vi "PIDController_EnableContinousInput.vi"(9 "MaxInput":dbl, 10 "MinInput":dbl, 11 "in PID_CONTROLLER":T1={"Kp"=0.0, "Ki"=0.0, "Kd"=0.0, "Period"=0.0, "Max_Integral"=0.0, "Min_Integral"=0.0, "Max_Input"=0.0, "Min_Input"=0.0, "Continuous"=FALSE, "PositionError"=0.0, "VelocityError"=0.0, "PrevError"=0.0, "TotalError"=0.0, "PositionTolerance"=0.0, "VelocityTolerance"=0.0, "SetPoint"=0.0, "Kf"=0.0, "Prev_Deriv"=0.0, "Prev_Deriv 2"=0.0, "DerivativeFilter"=FALSE, "Min_Output"=-9.99e+35, "Max_Output"=9.9e+35, "Prev_F_P"=0.0, "Prev_F_P_2"=0.0, "AntiWindupActive"=FALSE, "Measurement"=0.0, "IntegralZone"=9.9e+30} {"IntegralZone" format="%16_6e"; "Measurement" format="%16_6e"; "Prev_F_P_2" format="%16_6e"; "Prev_F_P" format="%16_6e"; "Max_Output" format="%16_6e"; "Min_Output" format="%16_6e"; "Prev_Deriv 2" format="%16_6e"; "Prev_Deriv" format="%16_6e"; "Kf" format="%16_6e"; "SetPoint" format="%16_6e"; "VelocityTolerance" format="%16_6e"; "PositionTolerance" format="%16_6e"; "TotalError" format="%16_6e"; "PrevError" format="%16_6e"; "VelocityError" format="%16_6e"; "PositionError" format="%16_6e"; "Min_Input" format="%16_6e"; "Max_Input" format="%16_6e"; "Min_Integral" format="%16_6e"; "Max_Integral" format="%16_6e"; "Period" format="%16_6e"; "Kd" format="%16_6e"; "Ki" format="%16_6e"; "Kp" format="%16_6e"}) -> (3 "out PID_CONTROLLER":T1={"Kp"=0.0, "Ki"=0.0, "Kd"=0.0, "Period"=0.0, "Max_Integral"=0.0, "Min_Integral"=0.0, "Max_Input"=0.0, "Min_Input"=0.0, "Continuous"=FALSE, "PositionError"=0.0, "VelocityError"=0.0, "PrevError"=0.0, "TotalError"=0.0, "PositionTolerance"=0.0, "VelocityTolerance"=0.0, "SetPoint"=0.0, "Kf"=0.0, "Prev_Deriv"=0.0, "Prev_Deriv 2"=0.0, "DerivativeFilter"=FALSE, "Min_Output"=-9.99e+35, "Max_Output"=9.9e+35, "Prev_F_P"=0.0, "Prev_F_P_2"=0.0, "AntiWindupActive"=FALSE, "Measurement"=0.0, "IntegralZone"=9.9e+30} {"IntegralZone" format="%16_6e"; "Measurement" format="%16_6e"; "Prev_F_P_2" format="%16_6e"; "Prev_F_P" format="%16_6e"; "Max_Output" format="%16_6e"; "Min_Output" format="%16_6e"; "Prev_Deriv 2" format="%16_6e"; "Prev_Deriv" format="%16_6e"; "Kf" format="%16_6e"; "SetPoint" format="%16_6e"; "VelocityTolerance" format="%16_6e"; "PositionTolerance" format="%16_6e"; "TotalError" format="%16_6e"; "PrevError" format="%16_6e"; "VelocityError" format="%16_6e"; "PositionError" format="%16_6e"; "Min_Input" format="%16_6e"; "Max_Input" format="%16_6e"; "Min_Integral" format="%16_6e"; "Max_Integral" format="%16_6e"; "Period" format="%16_6e"; "Kd" format="%16_6e"; "Ki" format="%16_6e"; "Kp" format="%16_6e"})   [LabVIEW 2019, in "Trajectory_Library.lvlib"]
doc: "Enables continuous input.\n \nRather then using the max and min input range as constraints, it considers them to be the same point and automatically calculates the shortest route to the setpoint.\n \nInputs:\n - PID_Controller -- PID_Controller data cluster\n - minimumInput -- The minimum value expected from the input.\n - maximumInput -- The maximum value expected from the input.\n\nOutputs:\n - PID_Controller -- Updated PID_Controller data cluster"
uses:
  Trajectory_Library.lvlib
  TypeDef/PID_CONTROLLER.ctl
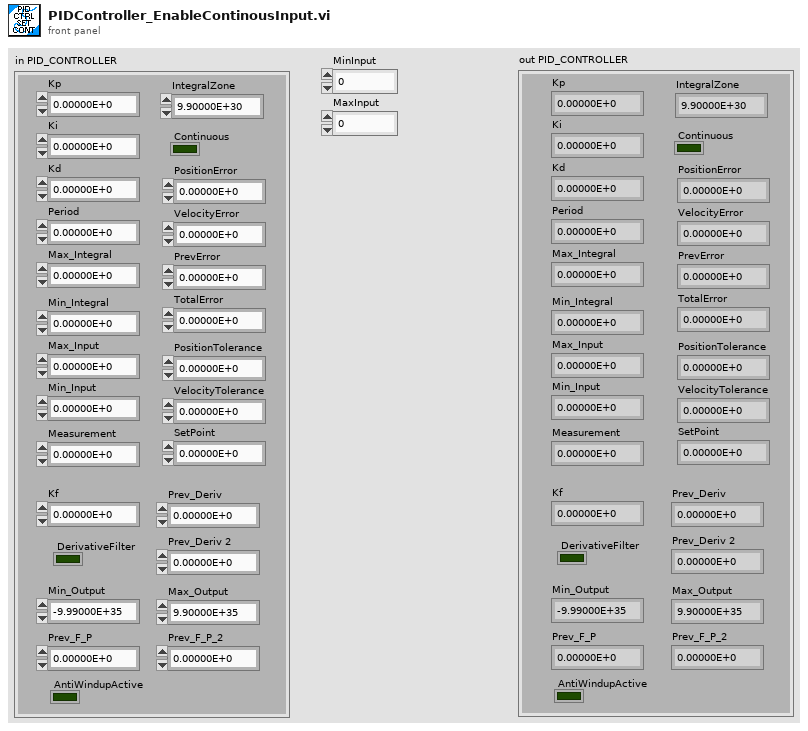
[diagram p1: front panel]
types:
  T1 = typedef "Trajectory_Library.lvlib/PID_CONTROLLER.ctl" = cluster{"Kp":dbl, "Ki":dbl, "Kd":dbl, "Period":dbl, "Max_Integral":dbl, "Min_Integral":dbl, "Max_Input":dbl, "Min_Input":dbl, "Continuous":bool, "PositionError":dbl, "VelocityError":dbl, "PrevError":dbl, "TotalError":dbl, "PositionTolerance":dbl, "VelocityTolerance":dbl, "SetPoint":dbl, "Kf":dbl, "Prev_Deriv":dbl, "Prev_Deriv 2":dbl, "DerivativeFilter":bool, "Min_Output":dbl, "Max_Output":dbl, "Prev_F_P":dbl, "Prev_F_P_2":dbl, "AntiWindupActive":bool, "Measurement":dbl, "IntegralZone":dbl}
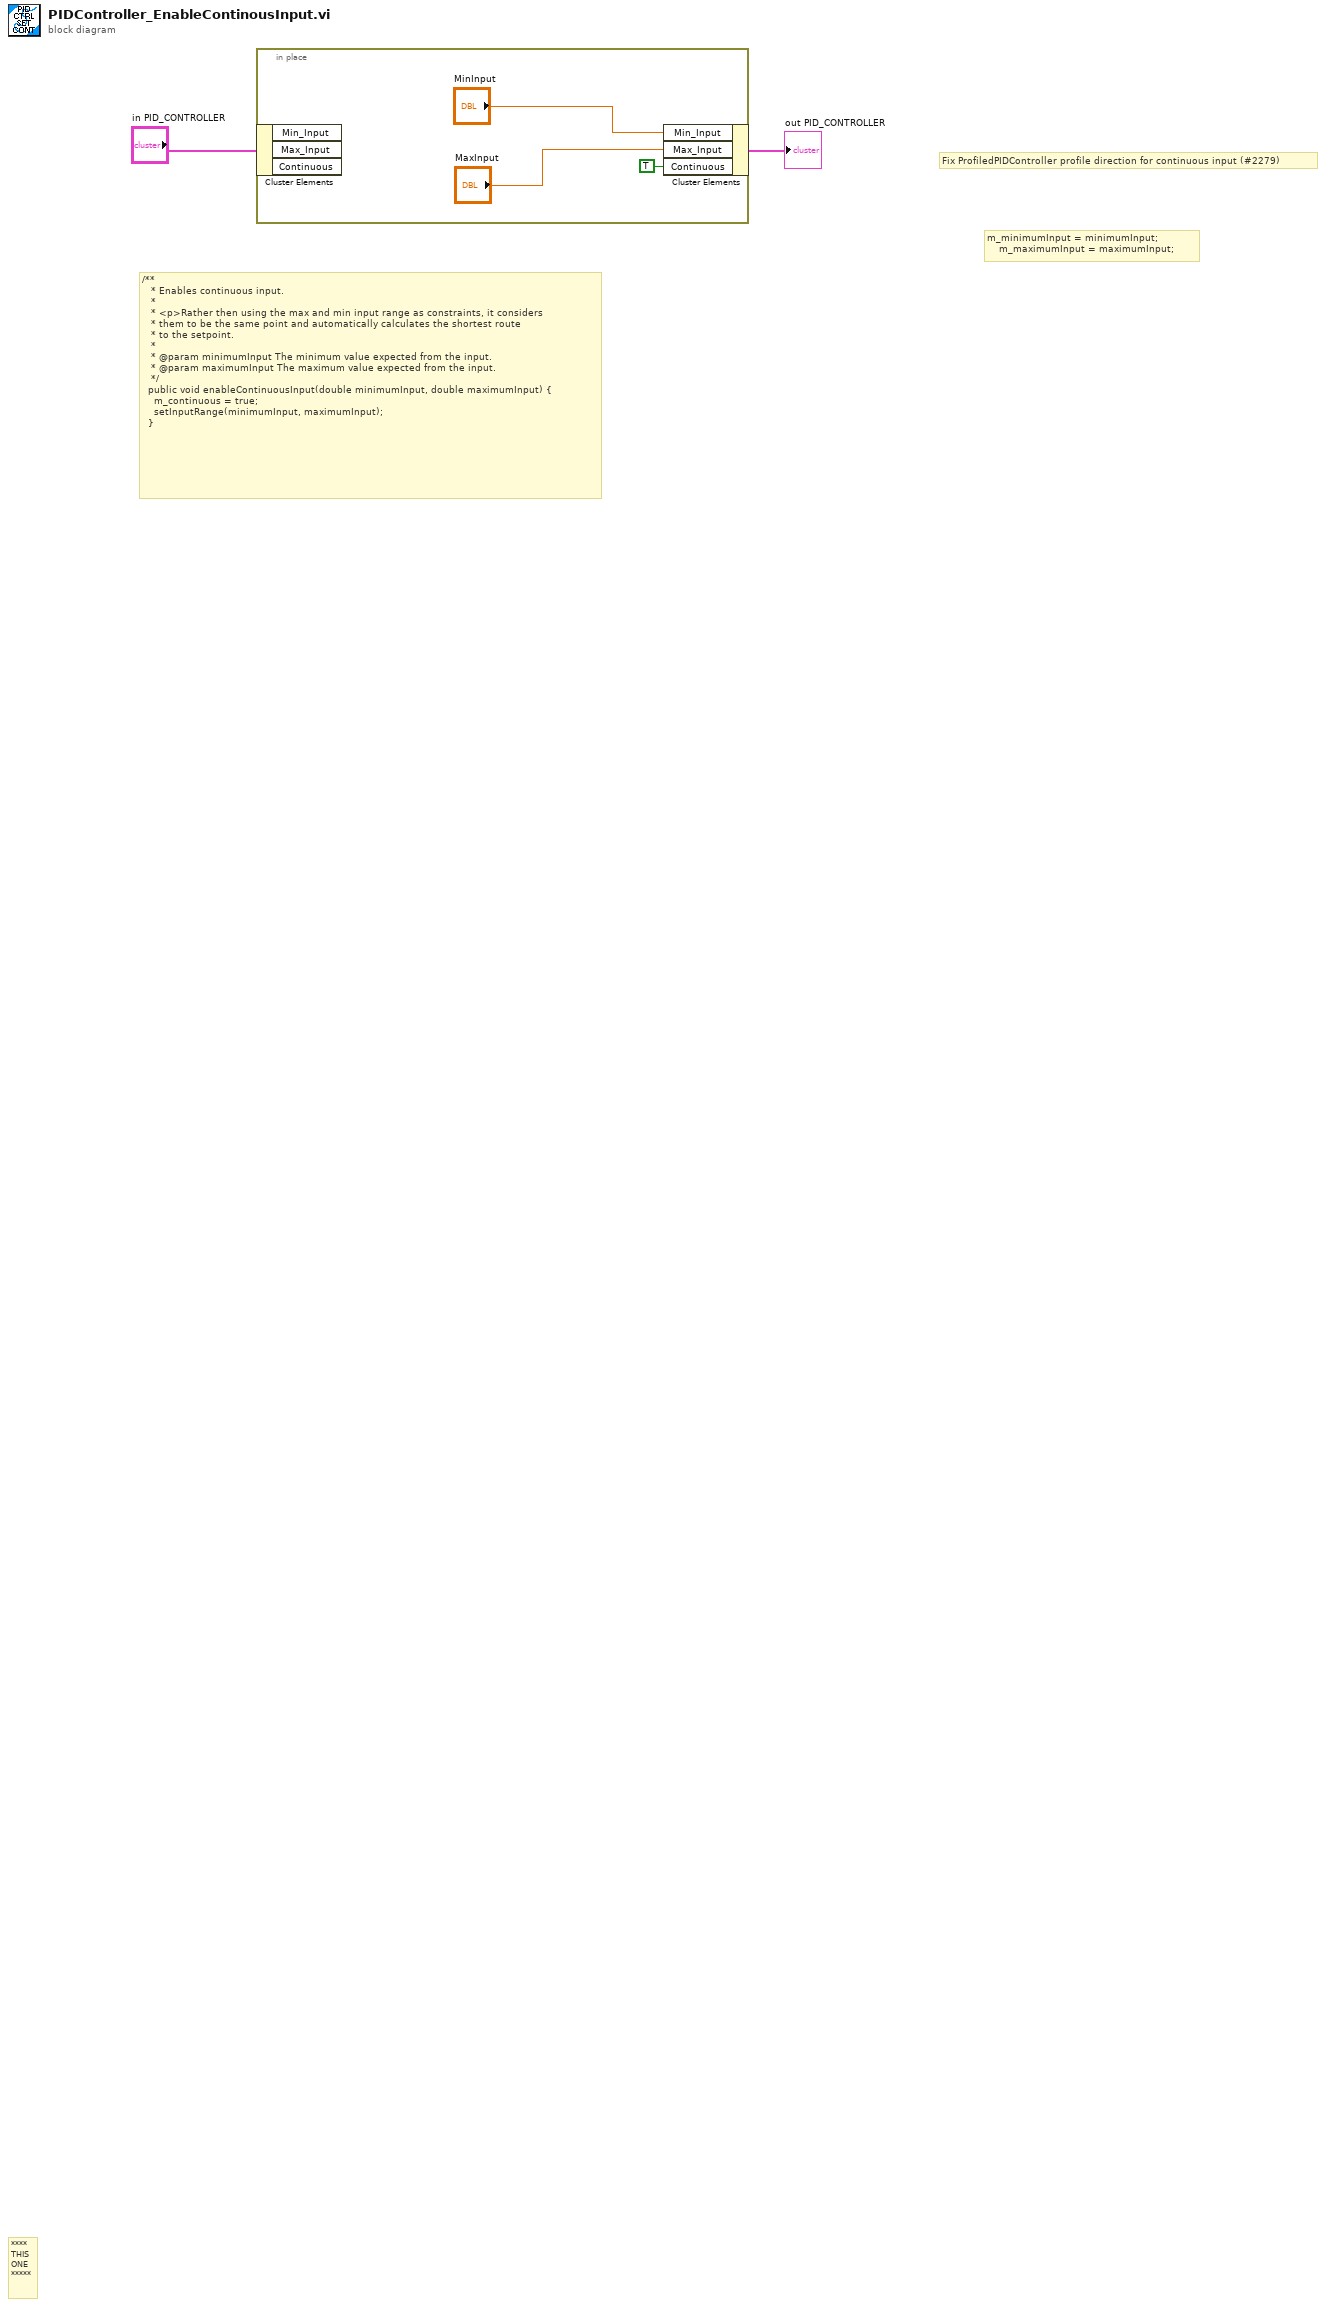
[diagram p0: block diagram]
diagram:
  # "m_minimumInput = minimumInput;\n    m_maximumInput = maximumInput;"
  # "Fix ProfiledPIDController profile direction for continuous input (#2279)"
  # "/**\n   * Enables continuous input.\n   *\n   * <p>Rather then using the max and min input range as constraints, it considers\n   * them to be the same point and automatically calculates the shortest route\n   * to the setpoint.\n   *\n   * @param minimumInput The minimum value expected from the input.\n   * @param maximumInput The maximum value expected from the input.\n   */\n  public void enableContinuousInput(double minimumInput, double maximumInput) {\n    m_continuous = true;\n    setInputRange(minimumInput, maximumInput);\n  }"
  # "****\nTHIS\nONE\n*****"
  n1 = in-place {
    n2 = in-place-cluster #1("in PID_CONTROLLER") -> ()  [unwired: 3 out]
    n3 = in-place-cluster #1("Min_Input"="MinInput", "Max_Input"="MaxInput", "Continuous"=TRUE) -> (→"out PID_CONTROLLER":T1)
  }
